vi "Set HW Interface Inputs.vi"(8 "error in (no error)":errorcluster, 9 "Digital Inputs":T1, 10 "Analog Inputs":T2, 11 "Hardware Interface in":refnum<class "Hardware Interface.lvclass">) -> (0 "error out":errorcluster, 3 "Hardware Interface out":refnum<class "Hardware Interface.lvclass">)   [LabVIEW 2013, in "Hardware Interface.lvclass"]
uses:
  Hardware Interface.lvclass
  DblArrayWithName.ctl
  BoolArrayWithName.ctl
  Hardware Interface.lvclass/Hardware Interface.ctl
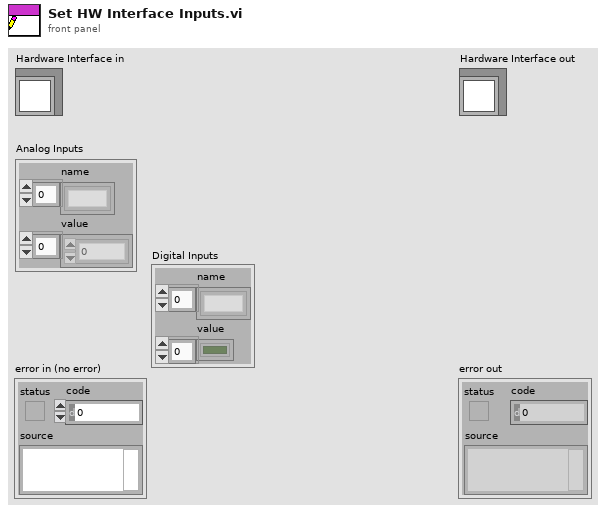
[diagram p1: front panel]
types:
  T1 = typedef "Hardware Interface.lvclass/BoolArrayWithName.ctl" = cluster{"name":string[], "value":bool[]}
  T2 = typedef "Hardware Interface.lvclass/DblArrayWithName.ctl" = cluster{"name":string[], "value":dbl[]}
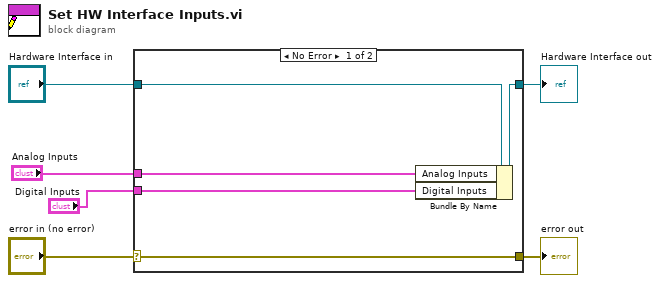
[diagram p0: block diagram]
diagram:
  n1 = case shown="No Error" "error in (no error)" {
    selector: "error in (no error)" -> [w11 w12]
    tunnel: [w11 w12] -> w5
    tunnel: [w9 w13] -> w3
    tunnel: "Hardware Interface in" -> [w10 w13]
    tunnel: "Analog Inputs" -> [w8 _]
    tunnel: "Digital Inputs" -> [w7 _]
    frame No Error {
      n2 = Bundle By Name(cluster=w10, "Analog Inputs"=w8, "Digital Inputs"=w7) -> (w9:refnum<class "Hardware Interface.lvclass">)
    }
    frame Error {
    }
  }
  "error out" <- w5
  "Hardware Interface out" <- w3
